vi "Read.vi"(0 "ILC ADC 2 in":refnum<class "ILC ADC 2.lvclass">, 5 "ILC In":refnum<class "ILC.lvclass">, 11 "error in (no error)":errorcluster) -> (4 "ILC ADC 2 out":refnum<class "ILC ADC 2.lvclass">, 6 "ILC Out":refnum<class "ILC.lvclass">, 8 "Value":dbl[unit], 10 "N":i32, 15 "error out":errorcluster)   [LabVIEW 2015, in "ILC ADC 2.lvclass"]
uses:
  ILC ADC 2.lvclass
  <userlib>/Common/ILC/ILC/ILC.lvclass
  <userlib>/Common/ILC/ILC/ILC.lvclass/ILC.ctl
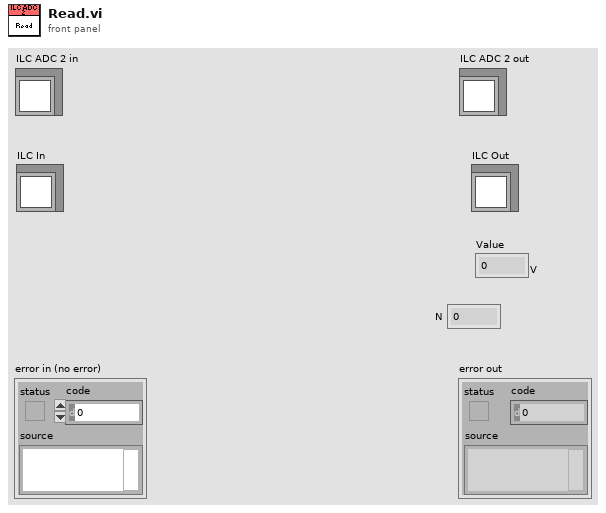
[diagram p1: front panel]
types:
  T1 = typedef "ILCCommon.lvlib/ILCTypedefs.lvlib/ADC Eng.ctl" = cluster{"Ch1":dbl[unit], "Ch2":dbl[unit], "Ch3":dbl[unit], "Ch4":dbl[unit]}
  T2 = typedef "ILCCommon.lvlib/ILCTypedefs.lvlib/Inputs.ctl" = cluster{"Input Channels":T3, "Limit Switches":T4, "Tachometer":u16, "SSI Encoder":i32, "ADC":T5}
  T3 = typedef "ILCCommon.lvlib/ILCConfiguration.lvlib/Input Channels.ctl" = enum16{"Channel 0", "3 Channels", "5 Channels"}
  T4 = typedef "ILCCommon.lvlib/ILCTypedefs.lvlib/Limit Switches.ctl" = cluster{"1":bool, "2":bool}
  T5 = typedef "ILCCommon.lvlib/ILCTypedefs.lvlib/ADC Raw.ctl" = cluster{"Ch0":i32, "Ch1":i32, "Ch2":i32, "Ch3":i32, "Ch4":i32}
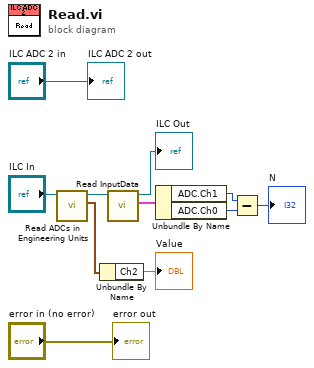
[diagram p0: block diagram]
diagram:
  n1 = call <userlib>:"Read ADCs in Engineering Units.vi"("ILC in"="ILC In") -> ("ADCs in Engineering Units"=w9:T1, "ILC out"=w4:refnum<class "ILC.lvclass">)  [unwired: 9 in]
  n2 = Unbundle By Name(w9) -> ("Ch2"=→"Value":dbl[unit])
  n3 = call <userlib>:"Read InputData.vi"("ILC in"=w4) -> ("InputData"=w5:T2, "ILC out"=→"ILC Out":refnum<class "ILC.lvclass">)  [unwired: 9 in]
  n4 = Unbundle By Name(w5) -> ("ADC.Ch1"=w2:i32, "ADC.Ch0"=w6:i32)
  n5 = Subtract(x=w2, y=w6) -> (x-y=→"N":i32)
  "error out" <- "error in (no error)"
  "ILC ADC 2 out" <- "ILC ADC 2 in"
